vi "Posix2Timestamp.vi"(5 "POSIX":dbl) -> (0 "date/time string":string, 1 "time tuple":T1, 2 "time stamp":timestamp format="%<%Y-%m-%dT%H:%M:%S %z %Z>T")   [LabVIEW 2020]
uses:
  <vilib>/Utility/miscctls.llb/LVDateTimeRec.ctl
panel:
  # "converts a POSIX timestamp (seconds since 1970-01-01 00:00:00) into LabVIEW timestamp format"
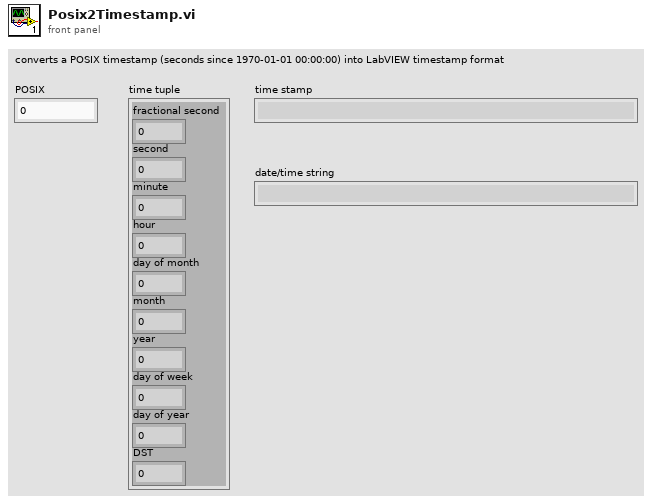
[diagram p1: front panel]
types:
  T1 = typedef "LVDateTimeRec.ctl" = cluster{"fractional second":dbl, "second":i32, "minute":i32, "hour":i32, "day of month":i32, "month":i32, "year":i32, "day of week":i32, "day of year":i32, "DST":i32}
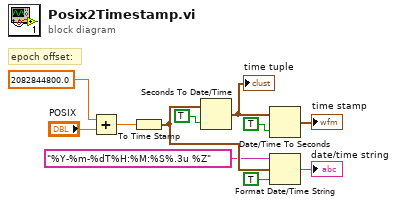
[diagram p0: block diagram]
diagram:
  # "epoch offset:"
  n1 = Add(x=2082844800.0, y="POSIX") -> (x+y=w11:dbl)
  n2 = To Time Stamp(1:w11) -> (0:w4:timestamp)
  n3 = Seconds To Date/Time(time stamp (now)=w4, to UTC (F)=TRUE) -> (date time rec=w5:T1)
  "time tuple" <- w5
  n4 = Date/Time To Seconds(1:TRUE ("is UTC (F)"), 2:w5) -> (0:→"time stamp":timestamp)
  n5 = Format Date/Time String(time format string (%c)="%Y-%m-%dT%H:%M:%S%.3u %Z", seconds (now)=w4, UTC format=TRUE) -> (date/time string=→"date/time string":string)
